vi "Hybrid Start Control Server.vi"() -> (0 "error out":errorcluster, 1 "dup reference":refnum<vi>)   [LabVIEW 2019]
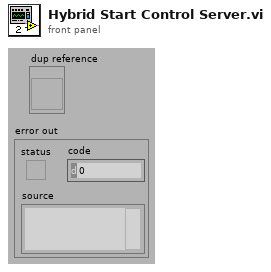
[diagram p1: front panel]
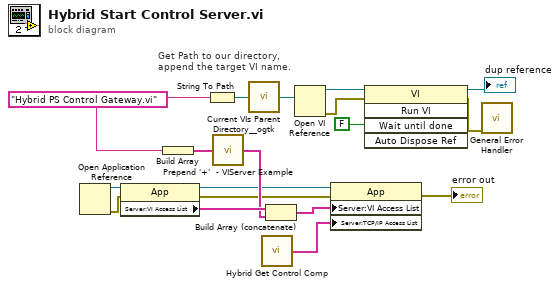
[diagram p0: block diagram]
diagram:
  w2 = "Hybrid PS Control Gateway.vi"
  # "Get Path to our directory,\nappend the target VI name."
  n1 = Open Application Reference() -> (0:w7:errorcluster, 3:w18:refnum<vi>)  [unwired: 4 in]
  n2 = property class="App"(reference=w18, error in=w7) -> (reference out=w8:refnum<vi>, error out=w9:errorcluster, "Server:VI Access List"=w12:string[])
  n3 = Build Array(w2) -> (w17:string[])
  n4 = String To Path(string=w2) -> (path=w4:path)
  n5 = call "Prepend '+'  - VIServer Example.vi"("list in"=w17) -> ("list out"=w11:string[])
  n6 = call <userlib>:"Current VIs Parent Directory__ogtk.vi"("Relative path (.)"=w4) -> ("Parent Directory (+ Relative)"=w3:path)  [unwired: 4 in]
  n7 = call "Hybrid Get Control Comp.vi"() -> ("Client 2"=w6:string[])
  n8 = Build Array (concatenate)(w12, w11) -> (w10:string[])
  n9 = Open VI Reference(vi path=w3) -> (vi reference=w16:refnum<vi>, error out=w1:errorcluster)  [unwired: 5 in]
  n10 = property class="App"(reference=w8, error in=w9, "Server:VI Access List"=w10, "Server:TCP/IP Access List"=w6) -> (error out=→"error out":errorcluster)  [unwired: 1 out]
  n11 = invoke class="VI" method="Run VI"(reference=w16, error in=w1, "Wait until done"=FALSE) -> (reference out=→"dup reference":refnum<vi>, error out=w14:errorcluster)  [unwired: 2 in, 3 out]
  n12 = call <vilib>:"General Error Handler.vi"("error in (no error)"=w14) -> ()  [unwired: 10 in, 5 out]
